vi "GetPuzzleData.vi"(8 "Error In":errorcluster) -> (0 "Error Out":errorcluster)   [LabVIEW 2020, in "AdventCode.lvclass"]
uses:
  AdventCode.lvclass
  <vilib>/httpClient/LabVIEWHTTPClient.lvlib
panel:
  out "body":string
  out "headers":string
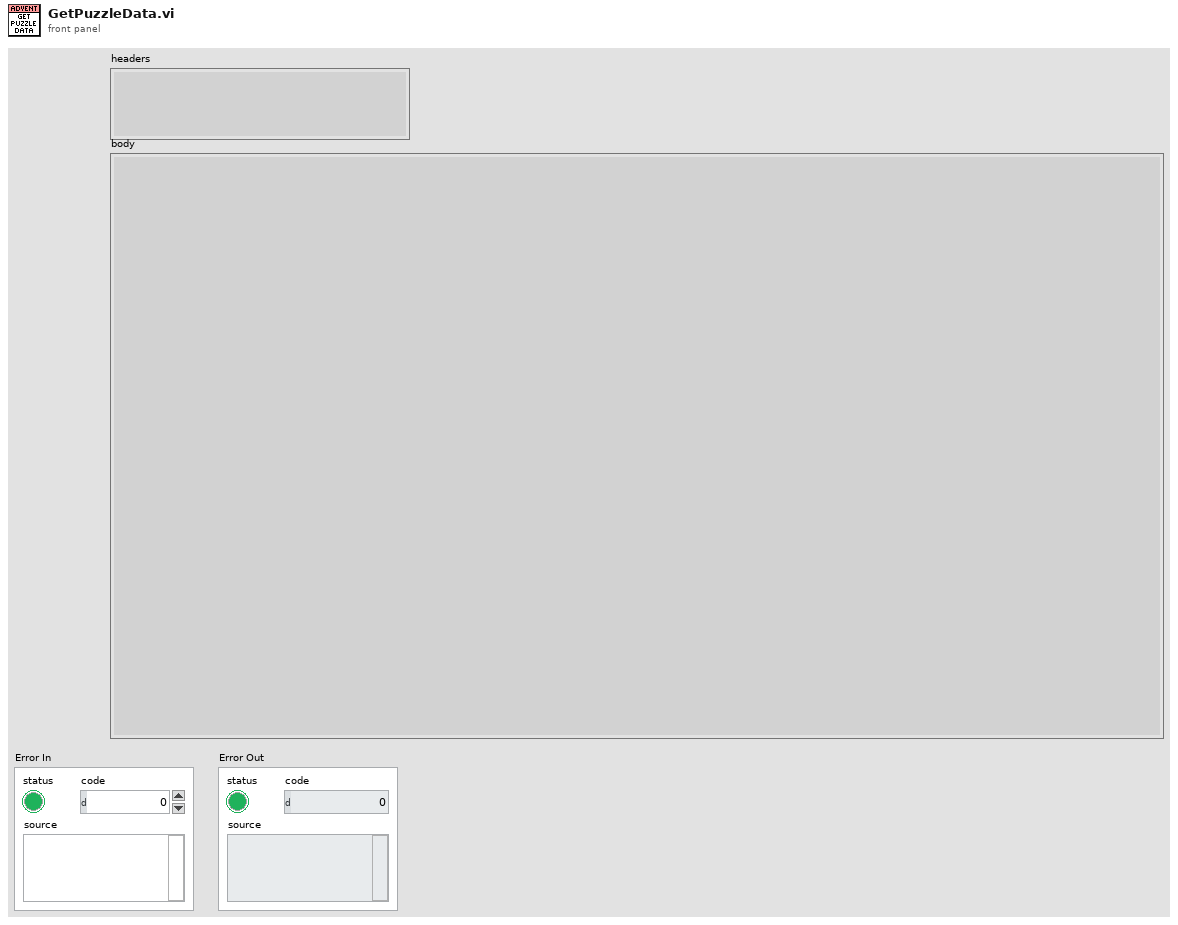
[diagram p1: front panel]
types:
  T1 = typedef "AdventCode.lvclass/ObjectAttributes.ctl" = cluster{"Year":i32, "Day":i32, "PuzzleData":string}
  T2 = typedef "Puzzle.lvclass/ObjectAttributes.ctl" = cluster{"Year":i32, "Day":i32, "PuzzleData":string}
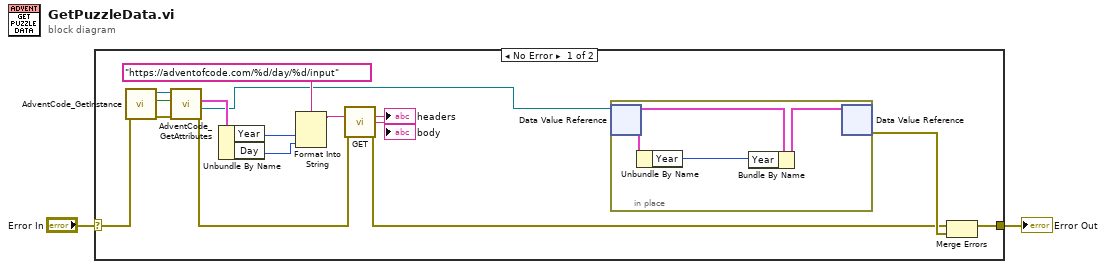
[diagram p0: block diagram]
diagram:
  n1 = case shown="No Error" "Error In" {
    selector: "Error In" -> [w17 w22]
    tunnel: [w18 w22] -> w1
    frame No Error {
      n2 = call "AdventCode_GetInstance.vi"("error in"=w17) -> ("error out"=w4:errorcluster, "NewObjectCreated"=w15:bool, "reference out"=w14:refnum<class "AdventCode.lvclass">)  [unwired: 6 in, 2 out]
      n3 = call "AdventCode_GetAttributes.vi"("error in (no error)"=w4, "OnlyGetDvrReference(False)"=w15, "reference in"=w14) -> ("error out"=w3:errorcluster, "DataRef"=w8:refnum<data-value>, "Data"=w13:T1)  [unwired: 5 in, 1 out]
      n4 = Unbundle By Name(w13) -> ("Year"=w11:i32, "Day"=w10:i32)
      n5 = Format Into String(format string="https://adventofcode.com/%d/day/%d/input", w11, w10) -> (resulting string=w9:string)  [unwired: 2 in, 1 out]
      n6 = call <vilib>:"GET.vi"("url"=w9, "error in (no error)"=w3) -> ("headers"=→"headers":string, "body"=→"body":string, "error out"=w5:errorcluster)  [unwired: 10 in, 1 out]
      n7 = in-place {
        n8 = in-place-dvr #1(w8) -> (w20:T2)  [unwired: 1 out]
        n9 = Unbundle By Name(w20) -> ("Year"=w19:i32)
        n10 = Bundle By Name(cluster=w20, "Year"=w19) -> (w21:T2)
        n11 = in-place-dvr #1(w21) -> (w16:errorcluster)  [unwired: 1 out]
      }
      n12 = Merge Errors(w5, w16) -> (w18:errorcluster)
    }
    frame Error {
    }
  }
  "Error Out" <- w1
